vi "PicoScopeospaStop.vi"(8 "error in (no error)":errorcluster, 11 "handle in":i16=16384) -> (0 "error out":errorcluster, 3 "handle out":i16)   [LabVIEW 2010]
doc: "This stops the device capturing data and should be called before retrieving data from the device."
uses:
  psospa.dll
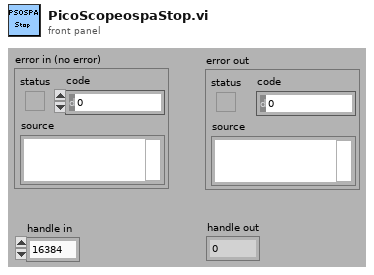
[diagram p1: front panel]
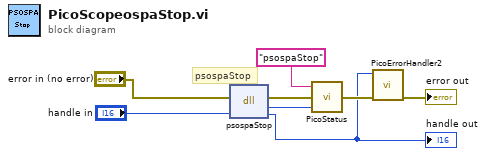
[diagram p0: block diagram]
diagram:
  # "psospaStop"
  n1 = dll-call lib="psospa.dll" fn="psospaStop"(error in="error in (no error)", "handle"="handle in") -> (error out=w8:errorcluster, "PICO_STATUS"=w7:u32, "handle"=w1:i16)  [unwired: 2 in, 1 out]
  "handle out" <- w1
  n2 = call "PicoStatus.vi"("PICO STATUS"=w7, "error in"=w8, "source"="psospaStop") -> ("error out"=w6:errorcluster)
  n3 = call "PicoErrorHandler2.vi"("error in (no error)"=w6, "handle In"=w1) -> ("error out"=→"error out":errorcluster)  [unwired: 9 in]
